vi "Switching Matrix.vi"(0 "Function":T2(tab), 1 "Setup Number \"n\"":i16 min=0 max=100 step=1, 2 "Data Format":T5(ring), 3 "SwitchMatrix Refnums":T6, 5 "VISA Resource Name":refnum<visa-resource-name>="GPIB0::18::INSTR", 7 "Set Switch Matrix":T3(array[cluster])=[{"Connections"=[FALSE, FALSE, FALSE, FALSE, FALSE, FALSE, FALSE, FALSE, FALSE, FALSE, FALSE, FALSE], "Connection Type"=enum."Disconnected"}, {"Connections"=[FALSE, FALSE, FALSE, FALSE, FALSE, FALSE, FALSE, FALSE, FALSE, FALSE, FALSE, FALSE], "Connection Type"=enum."Disconnected"}, {"Connections"=[FALSE, FALSE, FALSE, FALSE, FALSE, FALSE, FALSE, FALSE, FALSE, FALSE, FALSE, FALSE], "Connection Type"=enum."Disconnected"}, {"Connections"=[FALSE, FALSE, FALSE, FALSE, FALSE, FALSE, FALSE, FALSE, FALSE, FALSE, FALSE, FALSE], "Connection Type"=enum."Disconnected"}, {"Connections"=[FALSE, FALSE, FALSE, FALSE, FALSE, FALSE, FALSE, FALSE, FALSE, FALSE, FALSE, FALSE], "Connection Type"=enum."Disconnected"}, {"Connections"=[FALSE, FALSE, FALSE, FALSE, FALSE, FALSE, FALSE, FALSE, FALSE, FALSE, FALSE, FALSE], "Connection Type"=enum."Disconnected"}, {"Connections"=[FALSE, FALSE, FALSE, FALSE, FALSE, FALSE, FALSE, FALSE, FALSE, FALSE, FALSE, FALSE], "Connection Type"=enum."Disconnected"}, {"Connections"=[FALSE, FALSE, FALSE, FALSE, FALSE, FALSE, FALSE, FALSE, FALSE, FALSE, FALSE, FALSE], "Connection Type"=enum."Disconnected"}], 9 "Query":T4(ring), 11 "error in":errorcluster, 12 "Unit Number \"u\"":i16 min=0 max=4 step=1, 14 "Switchmatrix Notifications":T7) -> (6 "Message":string="\r\n", 8 "Get Switch Matrix":T3(array[cluster])=[{"Connections"=[FALSE, FALSE, FALSE, FALSE, FALSE, FALSE, FALSE, FALSE, FALSE, FALSE, FALSE, FALSE], "Connection Type"=enum."Disconnected"}, {"Connections"=[FALSE, FALSE, FALSE, FALSE, FALSE, FALSE, FALSE, FALSE, FALSE, FALSE, FALSE, FALSE], "Connection Type"=enum."Disconnected"}, {"Connections"=[FALSE, FALSE, FALSE, FALSE, FALSE, FALSE, FALSE, FALSE, FALSE, FALSE, FALSE, FALSE], "Connection Type"=enum."Disconnected"}, {"Connections"=[FALSE, FALSE, FALSE, FALSE, FALSE, FALSE, FALSE, FALSE, FALSE, FALSE, FALSE, FALSE], "Connection Type"=enum."Disconnected"}, {"Connections"=[FALSE, FALSE, FALSE, FALSE, FALSE, FALSE, FALSE, FALSE, FALSE, FALSE, FALSE, FALSE], "Connection Type"=enum."Disconnected"}, {"Connections"=[FALSE, FALSE, FALSE, FALSE, FALSE, FALSE, FALSE, FALSE, FALSE, FALSE, FALSE, FALSE], "Connection Type"=enum."Disconnected"}, {"Connections"=[FALSE, FALSE, FALSE, FALSE, FALSE, FALSE, FALSE, FALSE, FALSE, FALSE, FALSE, FALSE], "Connection Type"=enum."Disconnected"}, {"Connections"=[FALSE, FALSE, FALSE, FALSE, FALSE, FALSE, FALSE, FALSE, FALSE, FALSE, FALSE, FALSE], "Connection Type"=enum."Disconnected"}], 15 "error out":errorcluster)   [LabVIEW 2014]
uses:
  Switching Matrix Refnums.ctl
  Switching Matrix Notifiers.ctl
  support/Instrument Status.ctl
  support/Instrument Status State.ctl
  <vilib>/regexp/Match Regular Expression.xnode
  <instrlib>/Keithley 707A/Keithley 707A.lvlib
panel:
  out "Instrument Status":T1
  # "LICENSED MATERIALS – PROPERTY OF IBM\nCopyright IBM Corp. 2016,\nALL RIGHTS RESERVED"
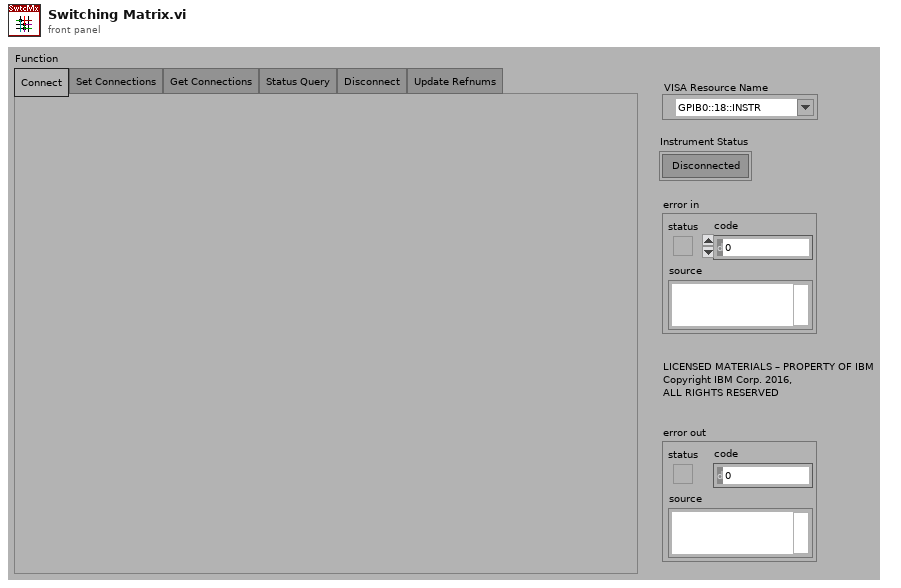
[diagram p1: front panel]
types:
  T1 = typedef "Instrument Status.ctl" = bool
  T2 = enum32{"Connect", "Set Connections", "Get Connections", "Status Query", "Disconnect", "Update Refnums"}
  T3 = cluster{"Connections":bool[], "Connection Type":enum16{"Disconnected", "Make - Break", "Break - Make"}}[]
  T4 = enum16{"Send Machine Status Word", "Send Error Status", "Output Setup \"n\" (0-100) with Current G Format", "Send RELAY STEP Pointer", "Send Number of Slaves", "Send Model Number of Each Card in Unit \"u\" (0-4)", "Send Relay Settling Time", "Send Digital Input", "Send RELAY TEST Input", "Set Data Format (G)"}
  T5 = enum16{"Full output format, all data sent in one talk", "Full output format, one row of one switching system per talk", "Inspect output format, all data sent in one talk", "Inspect output format, all data sent in one talk (again?)", "Condensed output format, all data sent in one talk", "Condensed output format, one switching system per talk", "Binary output format, all data sent in one talk", "Binary output format, one switching system per talk"}
  T6 = typedef "Switching Matrix Refnums.ctl" = cluster{"Connections":refnum<vi>, "Instrument Status":refnum<vi>}
  T7 = typedef "Switching Matrix Notifiers.ctl" = cluster{"Status":refnum<notifier>, "Instrument Data":refnum<notifier>, "Measurement":refnum<notifier>, "Exit":refnum<notifier>, "Ready":refnum<notifier>}
  T8 = cluster{"Connections":bool[], "Enum":enum16{"Disconnected", "Make - Break", "Break - Make"}}[]
  T9 = typedef "Instrument Status State.ctl" = enum16{"Unknown", "Idle", "Standby", "Configuring", "Measuring", "Moving", "Disconnected"}
  T10 = enum16{"Disconnected", "Make - Break", "Break - Make"}
  T11 = enum16{"Full output format, all data sent in one talk", "Full output format, one row of one switching system per talk", "Inspect output format, all data sent in one talk", "Inspect output format, one row of one switching system per talk", "Condensed output format, all data sent in one talk", "Condensed output format, one switching system per talk", "Binary output format, all data sent in one talk", "Binary output format, one switching system per talk"}
  T12 = cluster{"Connections":bool[], "Connection Type":enum16{"Disconnected", "Make - Break", "Break - Make"}}
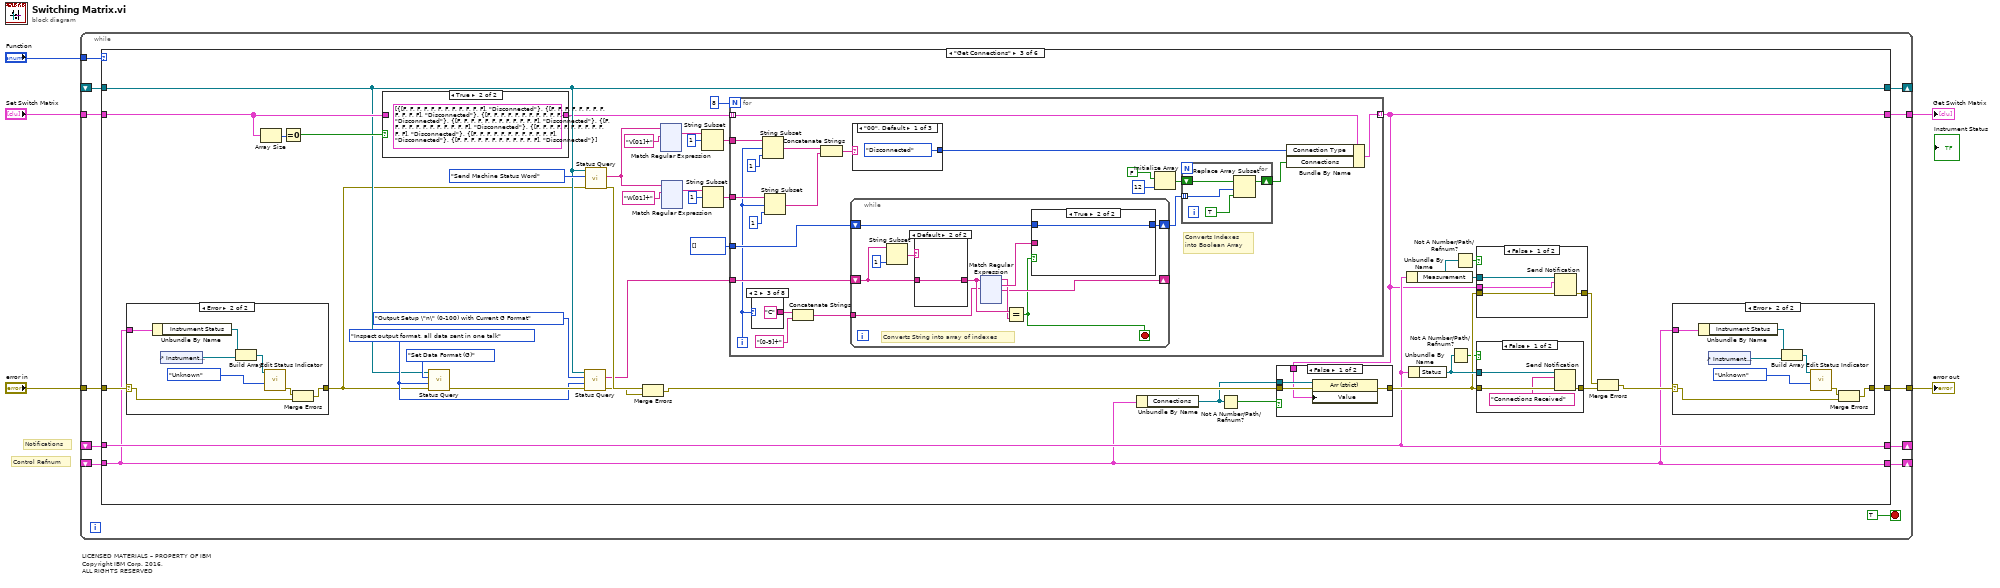
[diagram p0: block diagram]
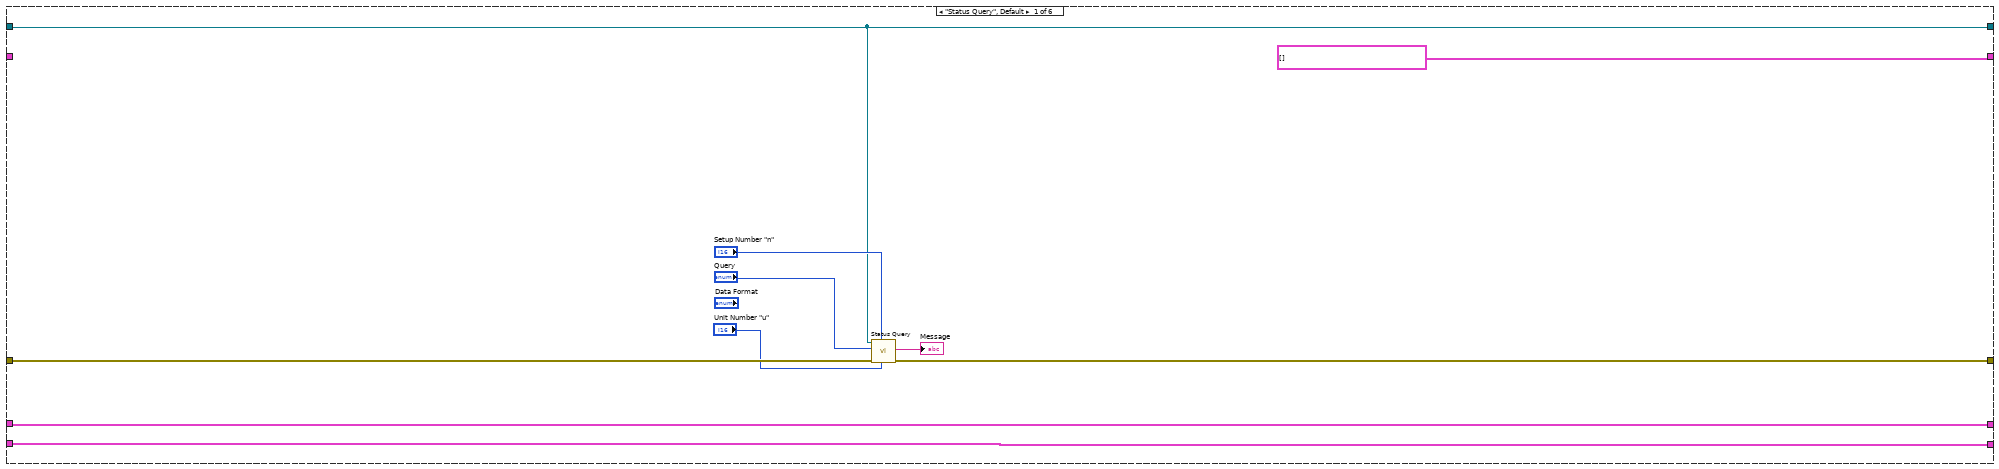
[diagram p2: hidden frame]
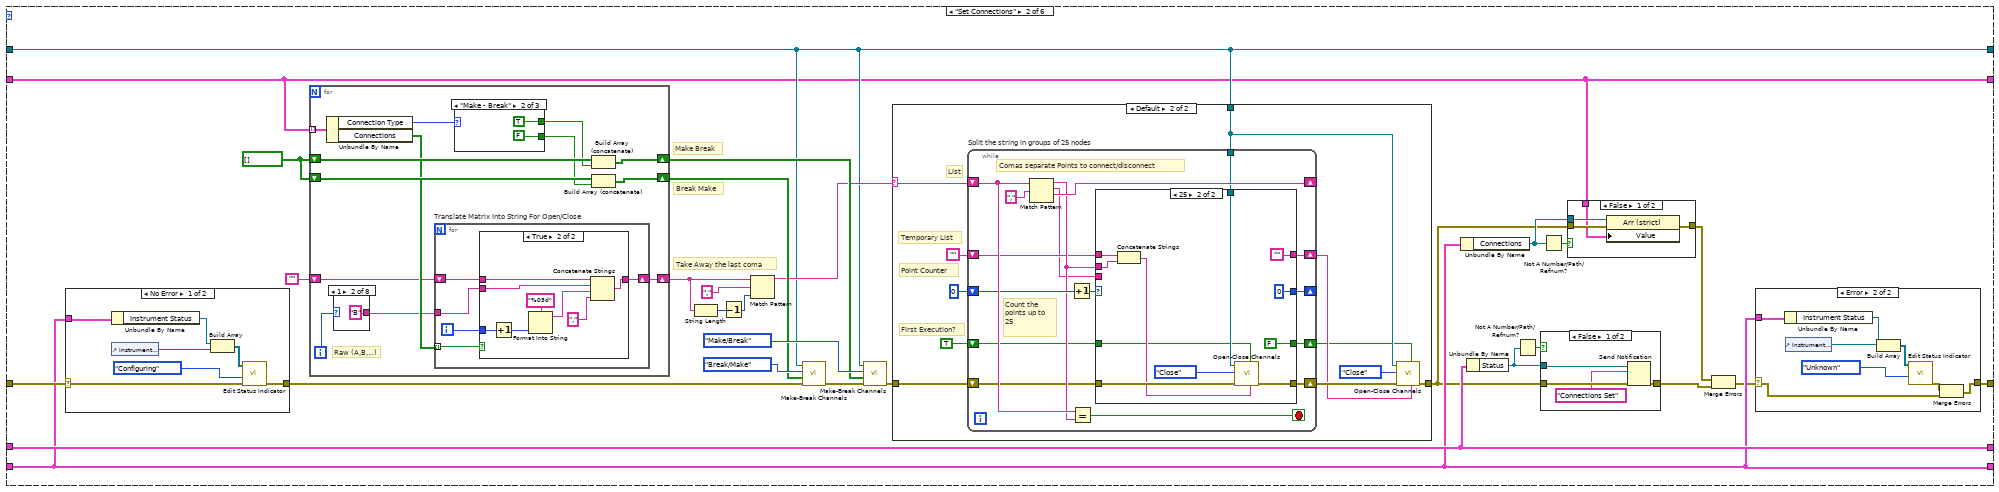
[diagram p3: hidden frame]
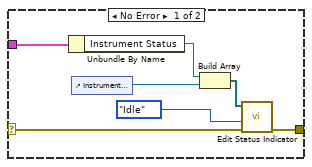
[diagram p5: hidden frame]
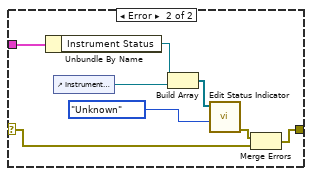
[diagram p6: hidden frame]
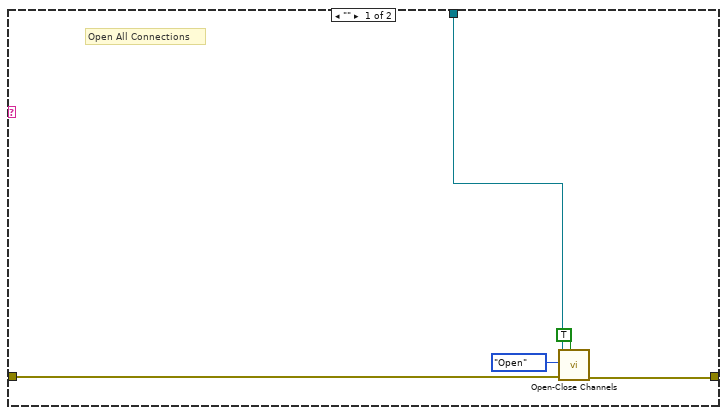
[diagram p8: hidden frame]
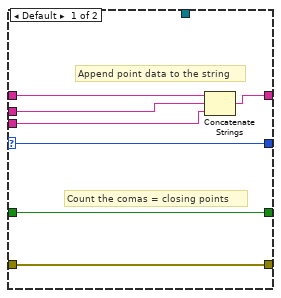
[diagram p9: hidden frame]
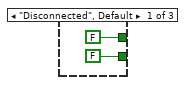
[diagram p10: hidden frame]
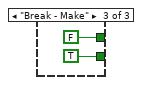
[diagram p11: hidden frame]
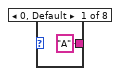
[diagram p12: hidden frame]
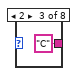
[diagram p13: hidden frame]
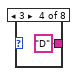
[diagram p14: hidden frame]
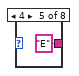
[diagram p15: hidden frame]
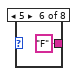
[diagram p16: hidden frame]
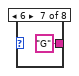
[diagram p17: hidden frame]
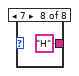
[diagram p18: hidden frame]
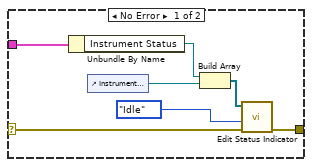
[diagram p20: hidden frame]
diagram:
  # "LICENSED MATERIALS – PROPERTY OF IBM\nCopyright IBM Corp. 2016,\nALL RIGHTS RESERVED"
  # "Control Refnum"
  # "Notifications"
  n1 = while {
    tunnel: "Function" -> [w17]
    tunnel: "error in" -> [w16]
    tunnel: [w15] -> w3
    tunnel: "Set Switch Matrix" -> [w13]
    shift-right: [w11] -> _
    shift-left: _ -> [w14]
    tunnel: [w10] -> w2
    shift-right: [w9] -> _
    shift-left: _ -> [w8]
    shift-right: [w7] -> _
    shift-left: _ -> [w6]
    stop <- TRUE stop-if-true
    n2 = case shown="\"Get Connections\"" w17 {
      tunnel: w16 -> [w27 w38 w190 w685 w718 w741]
      tunnel: [w26 w35 w189 w679 w709 w739] -> w15
      tunnel: w14 -> [w21 w42 w205 w683 _ w744]
      tunnel: w13 -> [_ w31 w207 _ _ _]
      tunnel: [w21 w42 w205 w683 w716 w744] -> w11
      tunnel: [T8 [] ("Get Switch Matrix") w31 w193 T8 [] ("Get Switch Matrix") T8 [] ("Get Switch Matrix") T8 [] ("Get Switch Matrix")] -> w10
      tunnel: [w19 w34 w187 w676 w708 "SwitchMatrix Refnums"] -> w9
      tunnel: w8 -> [w19 w34 w187 w676 w708 _]
      tunnel: w6 -> [w18 w41 w197 w680 w710 _]
      tunnel: [w18 w41 w197 w680 w710 "Switchmatrix Notifications"] -> w7
      frame "Status Query", Default {
        n3 = call <instrlib>:"Status Query.vi"("Unit Number \"u\""="Unit Number \"u\"", "Setup Number \"n\""="Setup Number \"n\"", "error in (no error)"=w27, "Query"="Query", "VISA Resource Name"=w21) -> ("error out"=w26:errorcluster, "Message"=→"Message":string)  [unwired: 1 in, 4 out]
      }
      frame "Set Connections" {
        w55 = bool[] []
        # "Break Make"
        # "Make Break"
        # "Take Away the last coma"
        n4 = case shown="No Error" w38 {
          selector: w38 -> [w81 w85]
          tunnel: [w80 w84] -> w37
          tunnel: w34 -> [w76 w86]
          frame No Error {
            n5 = Unbundle By Name(w76) -> ("Instrument Status"=w77:refnum<vi>)
            n6 = control-ref of="Instrument Status"() -> (w79:refnum<vi>)
            n7 = Build Array(w77, w79) -> (w78:refnum<vi>[])
            n8 = call "Edit Status Indicator.vi"("error in (no error)"=w81, "State"=Instrument_Status_State."Configuring", "Instrument Status Refnum"=w78) -> ("error out"=w80:errorcluster)  [unwired: 1 in, 7 out]
          }
          frame Error {
            n9 = Unbundle By Name(w86) -> ("Instrument Status"=w87:refnum<vi>)
            n10 = control-ref of="Instrument Status"() -> (w89:refnum<vi>)
            n11 = Build Array(w87, w89) -> (w88:refnum<vi>[])
            n12 = call "Edit Status Indicator.vi"("State"=Instrument_Status_State."Unknown", "Instrument Status Refnum"=w88) -> ("error out"=w83:errorcluster)  [unwired: 2 in, 7 out]
            n13 = Merge Errors(w83, w85) -> (w84:errorcluster)
          }
        }
        n14 = for {
          tunnel: w31 -> [w158] mode=indexing
          shift-right: [w154] -> w48
          shift-left: w55 -> [w157]
          shift-right: [w155] -> w49
          shift-left: w55 -> [w156]
          shift-right: [w149] -> w45
          shift-left: "" -> [w151]
          i -> [w152]
          # "Raw (A,B,...)"
          n15 = Unbundle By Name(w158) -> ("Connection Type"=w148:T10, "Connections"=w153:bool[])
          n16 = case shown="1" w152 {
            tunnel: ["A" ("y") "B" ("y") "C" ("y") "D" ("y") "E" ("y") "F" ("y") "G" ("y") "H" ("y")] -> w150
            frame 0, Default {
            }
            frame 1 {
            }
            frame 2 {
            }
            frame 3 {
            }
            frame 4 {
            }
            frame 5 {
            }
            frame 6 {
            }
            frame 7 {
            }
          }
          n17 = for "Translate Matrix Into String For Open/Close" {
            tunnel: w153 -> [w174] mode=indexing
            tunnel: w150 -> [w175]
            shift-right: [w176] -> w149
            shift-left: w151 -> [w177]
            i -> [w173]
            n18 = case shown="True" w174 {
              tunnel: w177 -> [w178 w186]
              tunnel: [w178 w185] -> w176
              tunnel: w175 -> [_ w184]
              tunnel: w173 -> [_ w183]
              frame False {
              }
              frame True {
                n19 = Increment(x=w183) -> (x+1=w179:i32)
                n20 = Format Into String(format string="%03d", w179) -> (resulting string=w181:string)  [unwired: 2 in, 1 out]
                n21 = Concatenate Strings(w186, w184, w181, "," ("string")) -> (w185:string)
              }
            }
          }
          n22 = case shown="\"Make - Break\"" w148 {
            tunnel: [FALSE TRUE FALSE] -> w147
            tunnel: [FALSE FALSE TRUE] -> w146
            frame "Disconnected", Default {
            }
            frame "Make - Break" {
            }
            frame "Break - Make" {
            }
          }
          n23 = Build Array (concatenate)(w157, w147) -> (w154:bool[])
          n24 = Build Array (concatenate)(w156, w146) -> (w155:bool[])
        }
        n25 = String Length(string=w45) -> (length=w47:i32)
        n26 = Decrement(x=w47) -> (x-1=w43:i32)
        n27 = Match Pattern(string=w45, regular expression=",", offset (0)=w43) -> (before substring=w44:string)  [unwired: 3 out]
        n28 = call <instrlib>:"Make-Break Channels.vi"("error in (no error)"=w37, "Raws"=w49, "Switching Order"=enum16{"Make/Break", "Break/Make"}."Break/Make", "VISA Resource Name"=w42) -> ("error out"=w54:errorcluster)  [unwired: 7 out]
        n29 = call <instrlib>:"Make-Break Channels.vi"("error in (no error)"=w54, "Raws"=w48, "Switching Order"=enum16{"Make/Break", "Break/Make"}."Make/Break", "VISA Resource Name"=w42) -> ("error out"=w53:errorcluster)  [unwired: 7 out]
        n30 = case shown="Default" w44 {
          selector: w44 -> [_ w102]
          tunnel: w53 -> [w100 w108]
          tunnel: [w99 w106] -> w28
          tunnel: w42 -> [w98 w104]
          frame "" {
            # "Open All Connections"
            n31 = call <instrlib>:"Open-Close Channels.vi"("Open Crosspoints"=TRUE ("Relay Closure Control"), "error in (no error)"=w100, "Function"=enum32{"Open", "Close"}."Open", "VISA Resource Name"=w98) -> ("error out"=w99:errorcluster)  [unwired: 3 in, 4 out]
          }
          frame Default {
            # "Point Counter"
            # "Temporary List"
            # "First Execution?"
            # "List"
            n32 = while "Split the string in groups of 25 nodes" {
              shift-right: [w124] -> _
              shift-left: w102 -> [w126]
              shift-right: [w118] -> w103
              shift-left: "" -> [w119]
              shift-right: [w121] -> _
              shift-left: 0 -> [w122]
              shift-right: [w116] -> w101
              shift-left: TRUE -> [w117]
              tunnel: w104 -> [w113]
              shift-right: [w114] -> w107
              shift-left: w108 -> [w115]
              stop <- w125 stop-if-true
              # "Comas separate Points to connect/disconnect"
              # "Count the points up to\n25"
              n33 = Match Pattern(string=w126, regular expression=",") -> (before substring=w120:string, match substring=w112:string, after substring=w124:string)  [unwired: 2 out]
              n34 = Increment(x=w122) -> (x+1=w123:i32)
              n35 = Equal?(x=w126, y=w120) -> (x = y?=w125:bool)
              n36 = case shown="25" w123 {
                selector: w123 -> [w134 _]
                tunnel: [w134 0] -> w121
                tunnel: w120 -> [w132 w143]
                tunnel: w119 -> [w133 w144]
                tunnel: [w131 ""] -> w118
                tunnel: w117 -> [w130 w135]
                tunnel: [w130 FALSE] -> w116
                tunnel: w115 -> [w129 w139]
                tunnel: [w129 w138] -> w114
                tunnel: w113 -> [_ w137]
                tunnel: w112 -> [w128 _]
                frame Default {
                  # "Count the comas = closing points"
                  # "Append point data to the string"
                  n37 = Concatenate Strings(w133, w132, w128) -> (w131:string)
                }
                frame 25 {
                  n38 = Concatenate Strings(w144, w143) -> (w136:string)
                  n39 = call <instrlib>:"Open-Close Channels.vi"("Crosspoints to Close"=w136, "Relay Closure Control"=w135, "error in (no error)"=w139, "Function"=enum32{"Open", "Close"}."Close", "VISA Resource Name"=w137) -> ("error out"=w138:errorcluster)  [unwired: 2 in, 4 out]
                }
              }
            }
            n40 = call <instrlib>:"Open-Close Channels.vi"("Crosspoints to Close"=w103, "Relay Closure Control"=w101, "error in (no error)"=w107, "Function"=enum32{"Open", "Close"}."Close", "VISA Resource Name"=w104) -> ("error out"=w106:errorcluster)  [unwired: 2 in, 4 out]
          }
        }
        n41 = Unbundle By Name(w34) -> ("Connections"=w33:refnum<vi>)
        n42 = Unbundle By Name(w41) -> ("Status"=w39:refnum<notifier>)
        n43 = Not A Number/Path/Refnum?(number/path/refnum=w39) -> (NaN/Path/Refnum?=w40:bool)
        n44 = case shown="False" w40 {
          tunnel: [w94 w95] -> w36
          tunnel: w39 -> [w93 _]
          tunnel: w28 -> [w92 w95]
          frame False {
            n45 = Send Notification(notification="Connections Set", notifier=w93, error in (no error)=w92) -> (error out=w94:errorcluster)  [unwired: 1 out]
          }
          frame True {
          }
        }
        n46 = Not A Number/Path/Refnum?(number/path/refnum=w33) -> (NaN/Path/Refnum?=w32:bool)
        n47 = case shown="False" w32 {
          tunnel: w28 -> [w59 w60]
          tunnel: [w58 w60] -> w29
          tunnel: w33 -> [w57 _]
          tunnel: w31 -> [w56 _]
          frame False {
            n48 = property class="Arr (strict)"(reference=w57, error in=w59, "Value"=w56) -> (error out=w58:errorcluster)  [unwired: 1 out]
          }
          frame True {
          }
        }
        n49 = Merge Errors(w29, w36) -> (w30:errorcluster)
        n50 = case shown="Error" w30 {
          selector: w30 -> [w66 w71]
          tunnel: [w65 w70] -> w35
          tunnel: w34 -> [w62 w72]
          frame No Error {
            n51 = Unbundle By Name(w62) -> ("Instrument Status"=w63:refnum<vi>)
            n52 = control-ref of="Instrument Status"() -> (w61:refnum<vi>)
            n53 = Build Array(w63, w61) -> (w64:refnum<vi>[])
            n54 = call "Edit Status Indicator.vi"("error in (no error)"=w66, "State"=Instrument_Status_State."Idle", "Instrument Status Refnum"=w64) -> ("error out"=w65:errorcluster)  [unwired: 1 in, 7 out]
          }
          frame Error {
            n55 = Unbundle By Name(w72) -> ("Instrument Status"=w73:refnum<vi>)
            n56 = control-ref of="Instrument Status"() -> (w68:refnum<vi>)
            n57 = Build Array(w73, w68) -> (w74:refnum<vi>[])
            n58 = call "Edit Status Indicator.vi"("State"=Instrument_Status_State."Unknown", "Instrument Status Refnum"=w74) -> ("error out"=w69:errorcluster)  [unwired: 2 in, 7 out]
            n59 = Merge Errors(w69, w71) -> (w70:errorcluster)
          }
        }
      }
      frame "Get Connections" {
        w211 = T11."Inspect output format, all data sent in one talk" ("Data Format")
        n60 = case shown="Error" w190 {
          selector: w190 -> [w248 w255]
          tunnel: [w247 w254] -> w191
          tunnel: w187 -> [w245 w252]
          frame No Error {
            n61 = Unbundle By Name(w245) -> ("Instrument Status"=w246:refnum<vi>)
            n62 = control-ref of="Instrument Status"() -> (w243:refnum<vi>)
            n63 = Build Array(w246, w243) -> (w244:refnum<vi>[])
            n64 = call "Edit Status Indicator.vi"("error in (no error)"=w248, "State"=Instrument_Status_State."Measuring", "Instrument Status Refnum"=w244) -> ("error out"=w247:errorcluster)  [unwired: 1 in, 7 out]
          }
          frame Error {
            n65 = Unbundle By Name(w252) -> ("Instrument Status"=w256:refnum<vi>)
            n66 = control-ref of="Instrument Status"() -> (w250:refnum<vi>)
            n67 = Build Array(w256, w250) -> (w251:refnum<vi>[])
            n68 = call "Edit Status Indicator.vi"("State"=Instrument_Status_State."Unknown", "Instrument Status Refnum"=w251) -> ("error out"=w253:errorcluster)  [unwired: 2 in, 7 out]
            n69 = Merge Errors(w253, w255) -> (w254:errorcluster)
          }
        }
        n70 = Array Size(array=w207) -> (size(s)=w208:i32)
        n71 = Equal To 0?(x=w208) -> (x = 0?=w206:bool)
        n72 = case shown="True" w206 {
          tunnel: w207 -> [w273 _]
          tunnel: [w273 T3 [{"Connections"=[FALSE, FALSE, FALSE, FALSE, FALSE, FALSE, FALSE, FALSE, FALSE, FALSE, FALSE, FALSE], "Connection Type"=enum."Disconnected"}, {"Connections"=[FALSE, FALSE, FALSE, FALSE, FALSE, FALSE, FALSE, FALSE, FALSE, FALSE, FALSE, FALSE], "Connection Type"=enum."Disconnected"}, {"Connections"=[FALSE, FALSE, FALSE, FALSE, FALSE, FALSE, FALSE, FALSE, FALSE, FALSE, FALSE, FALSE], "Connection Type"=enum."Disconnected"}, {"Connections"=[FALSE, FALSE, FALSE, FALSE, FALSE, FALSE, FALSE, FALSE, FALSE, FALSE, FALSE, FALSE], "Connection Type"=enum."Disconnected"}, {"Connections"=[FALSE, FALSE, FALSE, FALSE, FALSE, FALSE, FALSE, FALSE, FALSE, FALSE, FALSE, FALSE], "Connection Type"=enum."Disconnected"}, {"Connections"=[FALSE, FALSE, FALSE, FALSE, FALSE, FALSE, FALSE, FALSE, FALSE, FALSE, FALSE, FALSE], "Connection Type"=enum."Disconnected"}, {"Connections"=[FALSE, FALSE, FALSE, FALSE, FALSE, FALSE, FALSE, FALSE, FALSE, FALSE, FALSE, FALSE], "Connection Type"=enum."Disconnected"}, {"Connections"=[FALSE, FALSE, FALSE, FALSE, FALSE, FALSE, FALSE, FALSE, FALSE, FALSE, FALSE, FALSE], "Connection Type"=enum."Disconnected"}] ("Get Switch Matrix")] -> w204
          frame False {
          }
          frame True {
          }
        }
        n73 = call <instrlib>:"Status Query.vi"("error in (no error)"=w191, "Data Format"=w211, "Query"=T4."Set Data Format (G)", "VISA Resource Name"=w205) -> ("error out"=w226:errorcluster)  [unwired: 2 in, 5 out]
        n74 = call <instrlib>:"Status Query.vi"("error in (no error)"=w226, "Data Format"=w211, "Query"=T4."Output Setup \"n\" (0-100) with Current G Format", "VISA Resource Name"=w205) -> ("error out"=w224:errorcluster, "Message"=w210:string)  [unwired: 2 in, 4 out]
        n75 = call <instrlib>:"Status Query.vi"("error in (no error)"=w191, "Query"=T4."Send Machine Status Word", "VISA Resource Name"=w205) -> ("error out"=w225:errorcluster, "Message"=w214:string)  [unwired: 3 in, 4 out]
        n76 = Merge Errors(w225, w224) -> (w203:errorcluster)
        n77 = xnode "Match Regular Expression"("input string"=w214, "regular expression"="V[01]+") -> ("whole match"=w220:string)  [unwired: 2 in, 6 out]
        n78 = xnode "Match Regular Expression"("input string"=w214, "regular expression"="W[01]+") -> ("whole match"=w217:string)  [unwired: 2 in, 6 out]
        n79 = String Subset(string=w220, offset (0)=1) -> (substring=w222:string)  [unwired: 1 out]
        n80 = String Subset(string=w217, offset (0)=1) -> (substring=w215:string)  [unwired: 1 out]
        n81 = for {
          N: 8 -> [_]
          tunnel: w222 -> [w295]
          tunnel: w215 -> [w294]
          tunnel: [w291] -> w193 mode=indexing
          tunnel: w210 -> [w287]
          tunnel: i32[] [] -> [w290]
          tunnel: w204 -> [w279] mode=indexing
          i -> [w285]
          # "Converts Indexes \ninto Boolean Array"
          n82 = case shown="2" w285 {
            tunnel: ["A" ("y") "B" ("y") "C" ("y") "D" ("y") "E" ("y") "F" ("y") "G" ("y") "H" ("y")] -> w289
            frame 0, Default {
            }
            frame 1 {
            }
            frame 2 {
            }
            frame 3 {
            }
            frame 4 {
            }
            frame 5 {
            }
            frame 6 {
            }
            frame 7 {
            }
          }
          n83 = String Subset(string=w295, offset (0)=w285, length (rest)=1 ("length (rest)")) -> (substring=w277:string)
          n84 = String Subset(string=w294, offset (0)=w285, length (rest)=1 ("length (rest)")) -> (substring=w276:string)
          n85 = Concatenate Strings(w289, "[0-9]+" ("string")) -> (w286:string)
          n86 = Concatenate Strings(w277, w276) -> (w278:string)
          n87 = while {
            shift-right: [w315] -> _
            shift-left: w287 -> [w318]
            shift-right: [w311] -> w282
            shift-left: w290 -> [w313]
            tunnel: w286 -> [w312]
            stop <- w314 stop-if-true
            # "Converts String into array of indexes"
            n88 = String Subset(string=w318, length (rest)=1 ("length (rest)")) -> (substring=w317:string)  [unwired: 1 out]
            n89 = case shown="Default" w317 {
              tunnel: w318 -> [w331 w333]
              tunnel: [w332 w333] -> w320
              frame "," {
                n90 = String Subset(string=w331, offset (0)=1 ("length (rest)")) -> (substring=w332:string)  [unwired: 1 out]
              }
              frame Default {
              }
            }
            n91 = xnode "Match Regular Expression"("input string"=w320, "regular expression"=w312) -> ("before match"=w316:string, "whole match"=w321:string, "after match"=w315:string)  [unwired: 2 in, 4 out]
            n92 = Equal?(x=w320, y=w316) -> (x = y?=w314:bool)
            n93 = case shown="True" w314 {
              tunnel: w321 -> [w328 _]
              tunnel: w313 -> [w325 w329]
              tunnel: [w323 w329] -> w311
              frame False {
                n94 = String Subset(string=w328, offset (0)=1) -> (substring=w326:string)  [unwired: 1 out]
                n95 = Decimal String To Number(string=w326) -> (number=w324:i32)  [unwired: 3 out]
                n96 = Decrement(x=w324) -> (x-1=w322:i32)
                n97 = Build Array (concatenate)(w325, w322) -> (w323:i32[])
              }
              frame True {
              }
            }
          }
          n98 = case shown="\"00\", Default" w278 {
            tunnel: [T10."Disconnected" ("Connection Type") T10."Make - Break" ("Connection Type") T10."Break - Make" ("Connection Type")] -> w275
            frame "00", Default {
            }
            frame "10" {
            }
            frame "01" {
            }
          }
          n99 = Initialize Array(FALSE, 12 ("dimension size")) -> (w281:bool[])
          n100 = for {
            tunnel: w282 -> [w299] mode=indexing
            shift-right: [w301] -> w280
            shift-left: w281 -> [w302]
            n101 = Replace Array Subset(array=w302, new element=TRUE ("new element/subarray"), index=w299) -> (w301:bool[])
          }
          n102 = Bundle By Name(cluster=w279, "Connection Type"=w275, "Connections"=w280) -> (w291:T12)
        }
        n103 = Unbundle By Name(w187) -> ("Connections"=w201:refnum<vi>)
        n104 = Not A Number/Path/Refnum?(number/path/refnum=w201) -> (NaN/Path/Refnum?=w202:bool)
        n105 = case shown="False" w202 {
          tunnel: w203 -> [w271 w272]
          tunnel: [w270 w272] -> w198
          tunnel: w201 -> [w269 _]
          tunnel: w193 -> [w268 _]
          frame False {
            n106 = property class="Arr (strict)"(reference=w269, error in=w271, "Value"=w268) -> (error out=w270:errorcluster)  [unwired: 1 out]
          }
          frame True {
          }
        }
        n107 = Unbundle By Name(w197) -> ("Measurement"=w195:refnum<notifier>)
        n108 = Unbundle By Name(w197) -> ("Status"=w200:refnum<notifier>)
        n109 = Not A Number/Path/Refnum?(number/path/refnum=w200) -> (NaN/Path/Refnum?=w196:bool)
        n110 = Not A Number/Path/Refnum?(number/path/refnum=w195) -> (NaN/Path/Refnum?=w194:bool)
        n111 = case shown="False" w196 {
          tunnel: [w266 w267] -> w199
          tunnel: w200 -> [w265 _]
          tunnel: w198 -> [w264 w267]
          frame False {
            n112 = Send Notification(notification="Connections Received", notifier=w265, error in (no error)=w264) -> (error out=w266:errorcluster)  [unwired: 1 out]
          }
          frame True {
          }
        }
        n113 = case shown="False" w194 {
          tunnel: [w261 w262] -> w192
          tunnel: w195 -> [w260 _]
          tunnel: w198 -> [w259 w262]
          tunnel: w193 -> [w258 _]
          frame False {
            n114 = Send Notification(notification=w258, notifier=w260, error in (no error)=w259) -> (error out=w261:errorcluster)  [unwired: 1 out]
          }
          frame True {
          }
        }
        n115 = Merge Errors(w192, w199) -> (w188:errorcluster)
        n116 = case shown="Error" w188 {
          selector: w188 -> [w233 w239]
          tunnel: [w232 w238] -> w189
          tunnel: w187 -> [w229 w236]
          frame No Error {
            n117 = Unbundle By Name(w229) -> ("Instrument Status"=w230:refnum<vi>)
            n118 = control-ref of="Instrument Status"() -> (w228:refnum<vi>)
            n119 = Build Array(w230, w228) -> (w231:refnum<vi>[])
            n120 = call "Edit Status Indicator.vi"("error in (no error)"=w233, "State"=Instrument_Status_State."Idle", "Instrument Status Refnum"=w231) -> ("error out"=w232:errorcluster)  [unwired: 1 in, 7 out]
          }
          frame Error {
            n121 = Unbundle By Name(w236) -> ("Instrument Status"=w240:refnum<vi>)
            n122 = control-ref of="Instrument Status"() -> (w235:refnum<vi>)
            n123 = Build Array(w240, w235) -> (w241:refnum<vi>[])
            n124 = call "Edit Status Indicator.vi"("State"=Instrument_Status_State."Unknown", "Instrument Status Refnum"=w241) -> ("error out"=w237:errorcluster)  [unwired: 2 in, 7 out]
            n125 = Merge Errors(w237, w239) -> (w238:errorcluster)
          }
        }
      }
      frame "Disconnect" {
        n126 = call <instrlib>:"Close.vi"("error in (no error)"=w685, "VISA resource name"=w683) -> ("error out"=w678:errorcluster)  [unwired: 9 out]
        n127 = case shown="No Error" w678 {
          selector: w678 -> [w691 w697]
          tunnel: [w690 w696] -> w677
          tunnel: w676 -> [w687 w694]
          frame No Error {
            n128 = Unbundle By Name(w687) -> ("Instrument Status"=w688:refnum<vi>)
            n129 = control-ref of="Instrument Status"() -> (w686:refnum<vi>)
            n130 = Build Array(w688, w686) -> (w689:refnum<vi>[])
            n131 = call "Edit Status Indicator.vi"("error in (no error)"=w691, "State"=Instrument_Status_State."Disconnected", "Instrument Status Refnum"=w689) -> ("error out"=w690:errorcluster)  [unwired: 1 in, 7 out]
          }
          frame Error {
            n132 = Unbundle By Name(w694) -> ("Instrument Status"=w698:refnum<vi>)
            n133 = control-ref of="Instrument Status"() -> (w693:refnum<vi>)
            n134 = Build Array(w698, w693) -> (w699:refnum<vi>[])
            n135 = call "Edit Status Indicator.vi"("State"=Instrument_Status_State."Unknown", "Instrument Status Refnum"=w699) -> ("error out"=w695:errorcluster)  [unwired: 2 in, 7 out]
            n136 = Merge Errors(w695, w697) -> (w696:errorcluster)
          }
        }
        n137 = Unbundle By Name(w680) -> ("Status"=w682:refnum<notifier>)
        n138 = Not A Number/Path/Refnum?(number/path/refnum=w682) -> (NaN/Path/Refnum?=w681:bool)
        n139 = case shown="False" w681 {
          tunnel: w677 -> [w704 w705]
          tunnel: [w703 w705] -> w679
          tunnel: w682 -> [w702 _]
          frame False {
            n140 = Send Notification(notification="Disconnected", notifier=w702, error in (no error)=w704) -> (error out=w703:errorcluster)  [unwired: 1 out]
          }
          frame True {
          }
        }
      }
      frame "Connect" {
        n141 = call <instrlib>:"Initialize.vi"("error in (no error)"=w718, "Reset (True)"=TRUE, "ID Query (True)"=TRUE, "Keithley 707A VISA Resource"="VISA Resource Name") -> ("error out"=w707:errorcluster, "VISA resource name out"=w716:refnum<visa-resource-name>)  [unwired: 6 out]
        n142 = case shown="Error" w707 {
          selector: w707 -> [w724 w730]
          tunnel: [w723 w729] -> w706
          tunnel: w708 -> [w720 w727]
          frame No Error {
            n143 = Unbundle By Name(w720) -> ("Instrument Status"=w721:refnum<vi>)
            n144 = control-ref of="Instrument Status"() -> (w719:refnum<vi>)
            n145 = Build Array(w721, w719) -> (w722:refnum<vi>[])
            n146 = call "Edit Status Indicator.vi"("error in (no error)"=w724, "State"=Instrument_Status_State."Idle", "Instrument Status Refnum"=w722) -> ("error out"=w723:errorcluster)  [unwired: 1 in, 7 out]
          }
          frame Error {
            n147 = Unbundle By Name(w727) -> ("Instrument Status"=w731:refnum<vi>)
            n148 = control-ref of="Instrument Status"() -> (w726:refnum<vi>)
            n149 = Build Array(w731, w726) -> (w732:refnum<vi>[])
            n150 = call "Edit Status Indicator.vi"("State"=Instrument_Status_State."Unknown", "Instrument Status Refnum"=w732) -> ("error out"=w728:errorcluster)  [unwired: 2 in, 7 out]
            n151 = Merge Errors(w728, w730) -> (w729:errorcluster)
          }
        }
        n152 = Unbundle By Name(w710) -> ("Status"=w711:refnum<notifier>)
        n153 = Not A Number/Path/Refnum?(number/path/refnum=w711) -> (NaN/Path/Refnum?=w712:bool)
        n154 = case shown="False" w712 {
          tunnel: w711 -> [w737 _]
          tunnel: w706 -> [w736 w738]
          tunnel: [w735 w738] -> w709
          frame False {
            w734 = "Connected"  # Status
            n155 = Send Notification(notification=w734, notifier=w737, error in (no error)=w736) -> (error out=w735:errorcluster)  [unwired: 1 out]
          }
          frame True {
          }
        }
      }
      frame "Update Refnums" {
        n156 = Unbundle By Name("Switchmatrix Notifications") -> ("Status"=w742:refnum<notifier>)
        n157 = Not A Number/Path/Refnum?(number/path/refnum=w742) -> (NaN/Path/Refnum?=w743:bool)
        n158 = case shown="False" w743 {
          tunnel: w741 -> [w750 w751]
          tunnel: [w749 w751] -> w739
          tunnel: w742 -> [w748 _]
          frame False {
            n159 = Send Notification(notification="Refnums Updated", notifier=w748, error in (no error)=w750) -> (error out=w749:errorcluster)  [unwired: 1 out]
          }
          frame True {
          }
        }
      }
    }
  }
  "error out" <- w3
  "Get Switch Matrix" <- w2
